vi "Actor Core.vi"(8 "error in":errorcluster, 11 "Nested in":refnum<class "[V] Waveform.lvclass">) -> (0 "error out":errorcluster, 3 "Actor out":refnum<class "Actor.lvclass">)   [LabVIEW 2023, in "[V] Waveform.lvlib" / "[V] Waveform.lvclass"]
doc: "(<B>Filename</B>: Actor Framework.lvlib:Actor.lvclass:Actor Core.vi)\n\nReceives messages to the actor, reacts to them, and initiates any error handling that may shut the actor down.\n\nDescendant classes may override this VI to append parallel tasks for the actor to complete while it handles messages. Overrides use the Call Parent Method node."
uses:
  [V] Waveform.lvclass
  C:/Program Files (x86)/National Instruments/LabVIEW 2023/vi.lib/ActorFramework/Actor/Actor.lvclass
  <vilib>/ActorFramework/Actor/Actor.lvclass
  <vilib>/ActorFramework/Actor/Actor.lvclass/Actor.ctl
  <vilib>/ActorFramework/Message Enqueuer/Message Enqueuer.lvclass/Message Enqueuer.ctl
  [V] Waveform.lvclass/[V] Waveform.ctl
  <vilib>/ActorFramework/Message Enqueuer/Init from Existing Queue.vi
  <vilib>/ActorFramework/Message Enqueuer/Enqueue.vi
  <vilib>/ActorFramework/Stop Msg/Stop Msg.lvclass
  C:/Program Files (x86)/National Instruments/LabVIEW 2023/vi.lib/ActorFramework/Message/Message.lvclass
  <vilib>/ActorFramework/Message Priority Queue/Priority Enqueue.vi
  <vilib>/ActorFramework/Message Enqueuer/Message Enqueuer.lvclass
  D:/2_GitHub/LabVIEW-Wfm/[V] Waveform/[V] Waveform/[V] Waveform.lvclass
panel:
  out "coordinate":string
  in  "lock?":bool
  out "graph":waveform(dbl)[](graph) caption="标题"
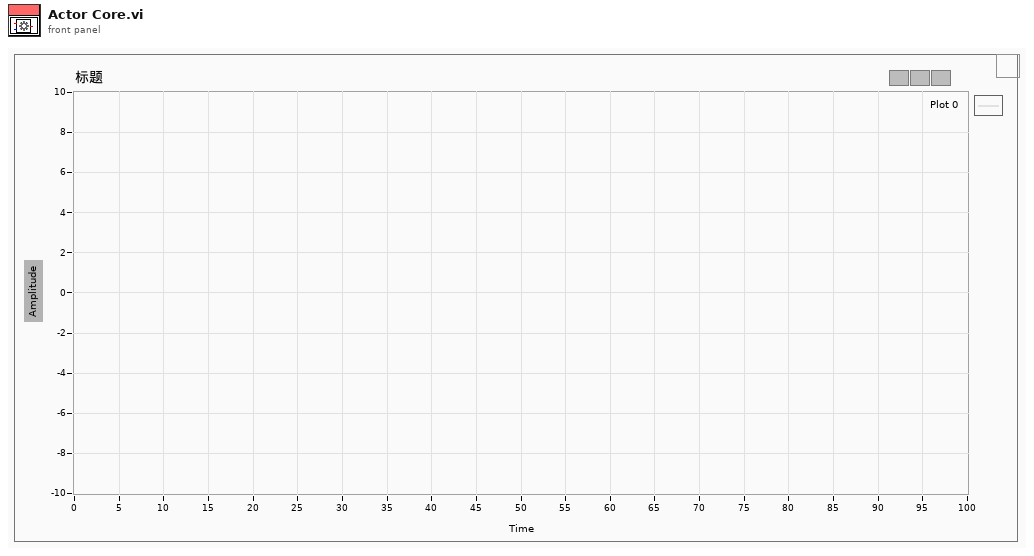
[diagram p1: front panel]
types:
  T1 = cluster{"stop":refnum<user-event>, "wave":refnum<user-event>}
  T2 = typedef "LVPoint32TypeDef.ctl" = cluster{"Horizontal":i32, "Vertical":i32}
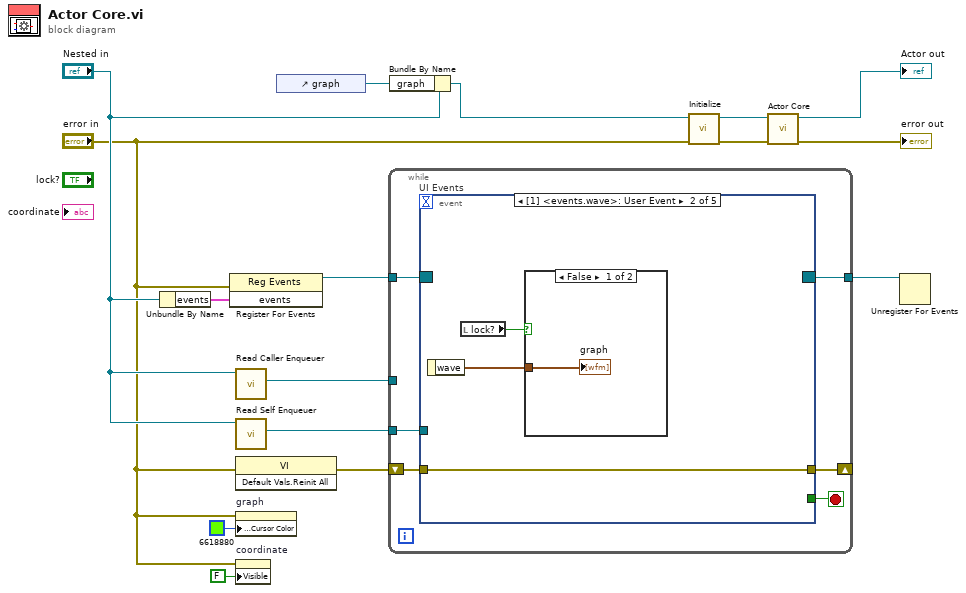
[diagram p0: block diagram]
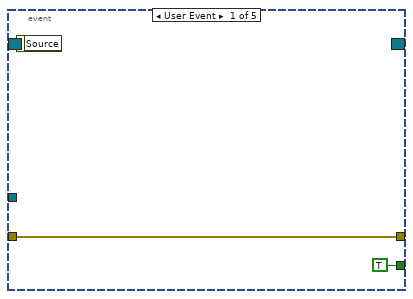
[diagram p2: hidden frame]
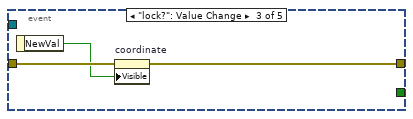
[diagram p4: hidden frame]
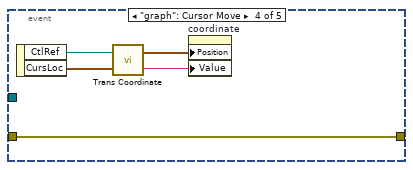
[diagram p5: hidden frame]
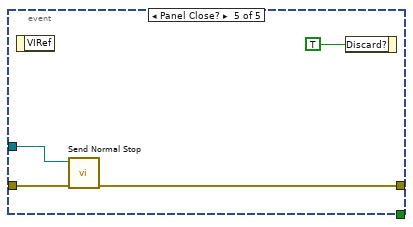
[diagram p6: hidden frame]
diagram:
  n1 = Unbundle By Name("Nested in") -> ("events"=w13:T1)
  n2 = register-events ("Main Register for Events")(error in="error in", w13) -> (reference out=w14:refnum<event-registration>)  [unwired: 1 in, 1 out]
  n3 = call <vilib>:"Read Caller Enqueuer.vi"("Actor"="Nested in") -> ("Caller Enqueuer"=w10:refnum<class "Message Enqueuer.lvclass">)  [unwired: 10 in]
  n4 = call <vilib>:"Read Self Enqueuer.vi"("Actor"="Nested in") -> ("Self Enqueuer"=w11:refnum<class "Message Enqueuer.lvclass">)  [unwired: 10 in]
  n5 = invoke class="VI" method="Default Vals.Reinit All"(error in="error in") -> (error out=w9:errorcluster)  [unwired: 2 in, 2 out]
  n6 = property on="graph" class="WFGraph (strict)"(error in="error in", "Cursor.Cursor Color"=u32 6618880) -> ()  [unwired: 1 in, 2 out]
  n7 = property on="coordinate" class="Str"(error in="error in", "Visible"=FALSE) -> ()  [unwired: 1 in, 2 out]
  n8 = control-ref of="graph"() -> (w4:refnum<vi>)
  n9 = while {
    tunnel: w14 -> [w22]
    tunnel: [w20] -> w12
    tunnel: w11 -> [w19]
    tunnel: w10 -> [_]
    shift-right: [w17] -> _
    shift-left: w9 -> [w18]
    stop <- w21 stop-if-true
    n10 = event "UI Events" shown="[1] <events.wave>: User Event" {
      selector: w22 -> [_ _ _ _ _]
      dyn-events: [_ _ _ _ _] -> w20
      timeout: _ -> [_ _ _ _ _]
      tunnel: [TRUE _ _ _ _] -> w21
      tunnel: w19 -> [_ _ _ _ w39]
      tunnel: w18 -> [w24 w26 w31 w32 w38]
      tunnel: [w24 w26 w29 w32 w37] -> w17
      event User Event {
        n11 = event-data() -> ()  [unwired: 1 in, 1 out]
      }
      event User Event {
        n12 = event-data() -> ("wave"=w27:waveform(dbl)[])  [unwired: 1 in]
        n13 = local read "lock?"() -> (w25:bool)
        n14 = case shown="False" w25 {
          tunnel: w27 -> [w28 _]
          frame False {
            "graph" <- w28
          }
          frame True {
          }
        }
      }
      event "lock?": Value Change {
        n15 = event-data() -> ("NewVal"=w30:bool)  [unwired: 1 in]
        n16 = property on="coordinate" class="Str"(error in=w31, "Visible"=w30) -> (error out=w29:errorcluster)  [unwired: 1 in, 1 out]
      }
      event "graph": Cursor Move {
        n17 = event-data() -> ("CtlRef"=w36:refnum<vi>, "CursLoc"=w35:cluster{"X":dbl, "Y":dbl})  [unwired: 1 in]
        n18 = call "Trans Coordinate.vi"("CursLoc"=w35, "CtlRef"=w36) -> ("coordinate"=w33:string, "Coords"=w34:T2)
        n19 = property on="coordinate" class="Str"("Position"=w34, "Value"=w33) -> ()  [unwired: 2 in, 2 out]
      }
      event Panel Close? {
        n20 = event-data() -> ()  [unwired: 1 in, 1 out]
        n21 = call <vilib>:"Send Normal Stop.vi"("error in (no error)"=w38, "Message Enqueuer"=w39) -> ("error out"=w37:errorcluster)  [unwired: 9 in]
        n22 = event-data("Discard?"=TRUE) -> ()  [unwired: 1 in, 1 out]
      }
    }
  }
  n23 = Bundle By Name(cluster="Nested in", "graph"=w4) -> (w5:refnum<class "[V] Waveform.lvclass">)
  n24 = call "Initialize.vi"("error in (no error)"="error in", "View Template in"=w5) -> ("error out"=w8:errorcluster, "View Template out"=w7:refnum<class "[V] Waveform.lvclass">)  [unwired: 8 in]
  n25 = call-parent "Actor Core.vi"("error in"=w8, "Actor in"=w7) -> ("error out"=→"error out":errorcluster, "Actor out"=→"Actor out":refnum<class "Actor.lvclass">)  [unwired: 8 in]
  n26 = Unregister For Events(event registration refnum=w12) -> ()  [unwired: 1 in, 1 out]
